vi "Config_LoadCreate.vi"(7 "Config In":path, 8 "error In":errorcluster, 10 "Configuration Cluster":T2={"General"={"Config.ini"=path "", "Default Logging Path"=path ""}, "Hardware"={"Global T VAR"="", "Global B VAR"="", "VISAS"={"GEN COM"="", "SCOPE COM"="", "VNA COM"=""}}, "Operation"={"Operation Mode"=enum."Idle-Off", "Status"="", "NewLog?"=FALSE, "OvenWarn"=FALSE, "Scope Settings"={"TimeBase"=0.0, "VerticalScale"=4.0}}}, 11 "?":T1) -> (0 "error out":errorcluster, 2 "Configuration Cluster Out":T2={"General"={"Config.ini"=path "", "Default Logging Path"=path ""}, "Hardware"={"Global T VAR"="", "Global B VAR"="", "VISAS"={"GEN COM"="", "SCOPE COM"="", "VNA COM"=""}}, "Operation"={"Operation Mode"=enum."Idle-Off", "Status"="", "NewLog?"=FALSE, "OvenWarn"=FALSE, "Scope Settings"={"TimeBase"=0.0, "VerticalScale"=4.0}}}, 3 "?":T1)   [LabVIEW 2021]
uses:
  Config_Cluster.ctl
  Mode_Enum.ctl
  VISAS.ctl
  <vilib>/Utility/config.llb/Read Key (Path).vi
  <vilib>/Utility/config.llb/NI_LVConfig.lvlib
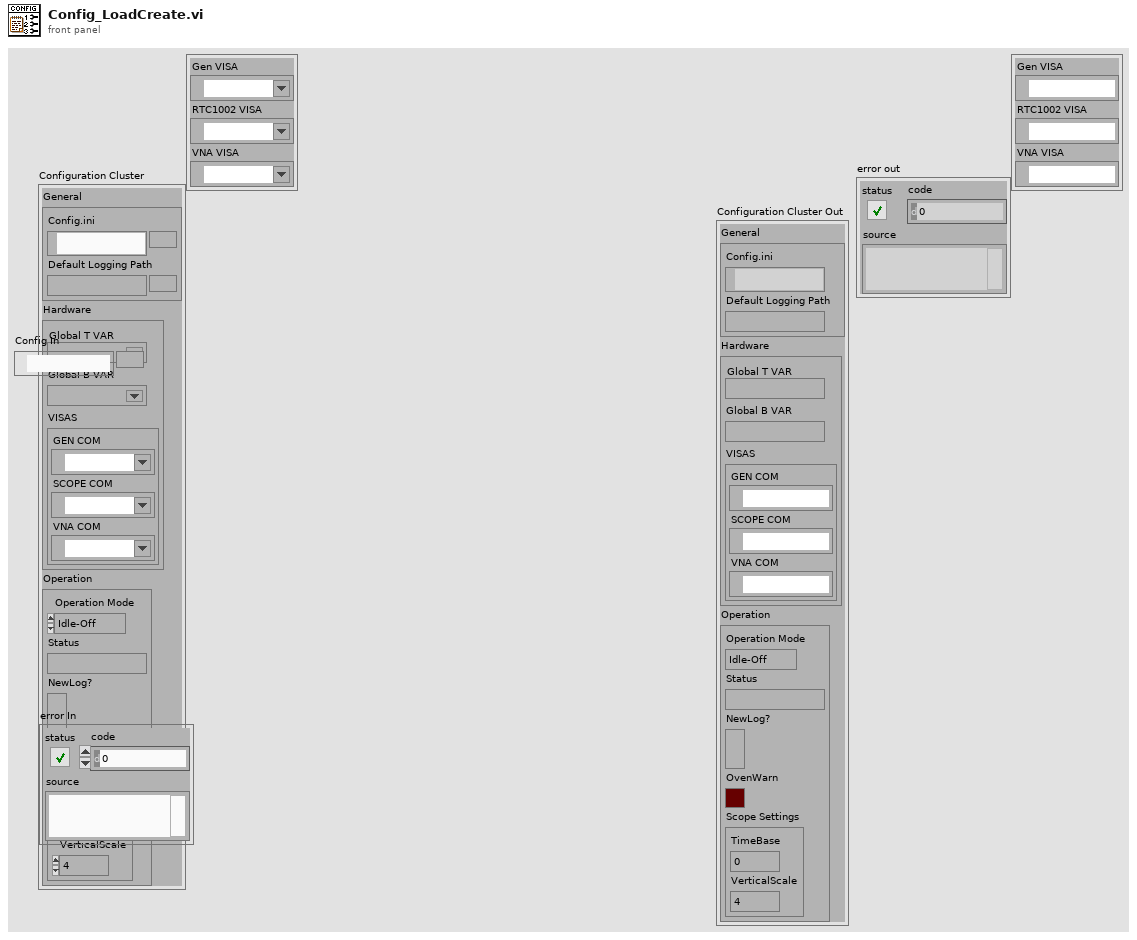
[diagram p1: front panel]
types:
  T1 = typedef "VISAS.ctl" = cluster{"Gen VISA":refnum<visa-resource-name>, "RTC1002 VISA":refnum<visa-resource-name>, "VNA VISA":refnum<visa-resource-name>}
  T2 = typedef "Config_Cluster.ctl" = cluster{"General":cluster{"Config.ini":path, "Default Logging Path":path}, "Hardware":cluster{"Global T VAR":refnum<k21>, "Global B VAR":refnum<k21>, "VISAS":cluster{"GEN COM":refnum<visa-resource-name>, "SCOPE COM":refnum<visa-resource-name>, "VNA COM":refnum<visa-resource-name>}}, "Operation":cluster{"Operation Mode":T3, "Status":string, "NewLog?":bool, "OvenWarn":bool, "Scope Settings":cluster{"TimeBase":dbl, "VerticalScale":dbl}}}
  T3 = typedef "Mode_Enum.ctl" = enum16{"OvenNRDY", "Logging", "Idle-Off", "Idle"}
  T4 = typedef "NI_LVConfig.lvlib/Config Data RefNum.ctl" = refnum<k1>
  T5 = cluster{"GEN COM":refnum<visa-resource-name>, "SCOPE COM":refnum<visa-resource-name>, "VNA COM":refnum<visa-resource-name>}
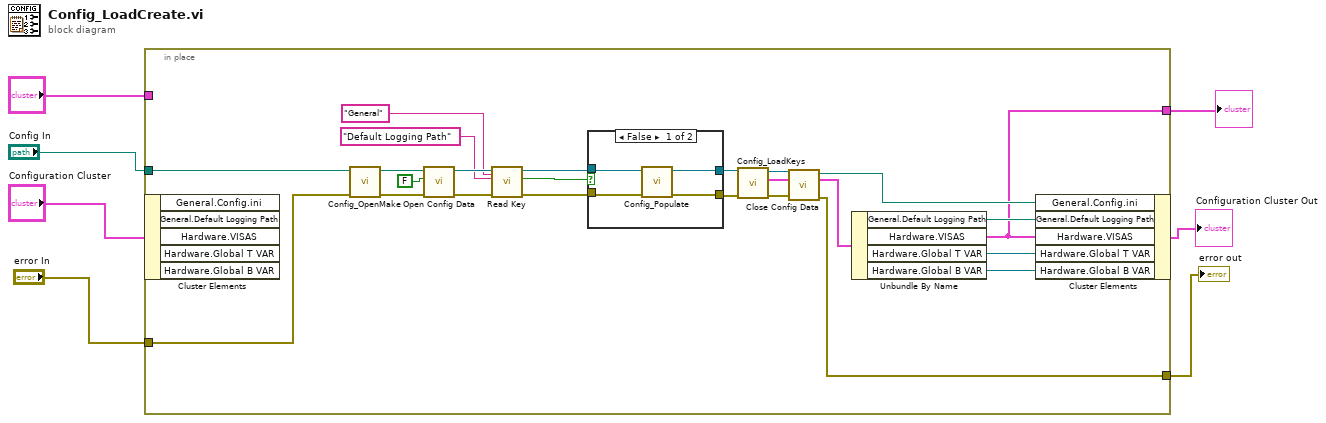
[diagram p0: block diagram]
diagram:
  n1 = in-place {
    in-place-border: "error In" -> [w29]
    in-place-border: "Config In" -> [w30]
    in-place-border: [w11] -> w1
    in-place-border: [w10] -> w3
    in-place-border: "?" -> [_]
    n2 = in-place-cluster #1("Configuration Cluster") -> ()  [unwired: 5 out]
    n3 = call "Config_OpenMake.vi"("error in (no error)"=w29, "Config Path"=w30) -> ("error out"=w26:errorcluster, "File Path"=w28:path)  [unwired: 8 in]
    n4 = call <vilib>:"Open Config Data.vi"("error in (no error)"=w26, "create file if necessary (T)"=FALSE, "configuration file path"=w28) -> ("error out"=w24:errorcluster, "refnum"=w25:T4)  [unwired: 6 in, 1 out]
    n5 = call-poly <vilib>:"Read Key.vi"("section"="General", "error in (no error)"=w24, "key"="Default Logging Path", "refnum"=w25) -> ("error out"=w20:errorcluster, "found?"=w19:bool, "refnum out"=w21:T4)  [unwired: 4 in, 1 out]
    n6 = case shown="False" w19 {
      tunnel: w20 -> [w33 w35]
      tunnel: w21 -> [w34 w36]
      tunnel: [w32 w35] -> w15
      tunnel: [w31 w36] -> w17
      frame False {
        n7 = call "Config_Populate.vi"("error in (no error)"=w33, "Config Ref In"=w34) -> ("error out"=w32:errorcluster, "refnum out"=w31:T4)  [unwired: 8 in]
      }
      frame True {
      }
    }
    n8 = call "Config_LoadKeys.vi"("error in (no error)"=w15, "Config In"=w17) -> ("error out"=w14:errorcluster, "output cluster"=w13:T2, "refnum out"=w16:T4)  [unwired: 7 in]
    n9 = call <vilib>:"Close Config Data.vi"("error in (no error)"=w14, "refnum"=w16) -> ("error out"=w10:errorcluster, "file path"=w18:path)  [unwired: 8 in]
    n10 = Unbundle By Name(w13) -> ("General.Default Logging Path"=w12:path, "Hardware.VISAS"=w11:T5, "Hardware.Global T VAR"=w9:refnum<k21>, "Hardware.Global B VAR"=w8:refnum<k21>)
    n11 = in-place-cluster #1("General.Config.ini"=w18, "General.Default Logging Path"=w12, "Hardware.VISAS"=w11, "Hardware.Global T VAR"=w9, "Hardware.Global B VAR"=w8) -> (→"Configuration Cluster Out":T2)
  }
  "error out" <- w3
  "?" <- w1
